vi "StartOrEnd.vi"(5 "Invert?":bool, 7 "StartOrEnd":string(combo), 10 "y":string, 11 "x":string) -> (2 "Equal?":bool)   [LabVIEW 2018]
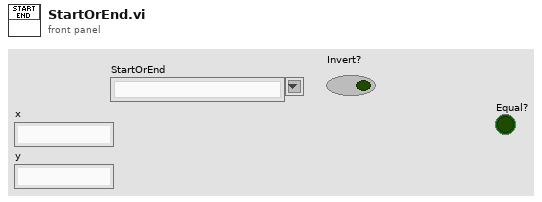
[diagram p1: front panel]
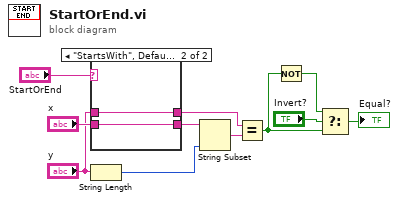
[diagram p0: block diagram]
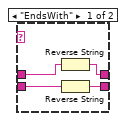
[diagram p2: hidden frame]
diagram:
  n1 = case shown="\"StartsWith\", Default" "StartOrEnd" {
    tunnel: [w14 w17] -> w5
    tunnel: "x" -> [w15 w17]
    tunnel: [w12 w16] -> w3
    tunnel: "y" -> [w13 w16]
    frame "EndsWith" {
      n2 = Reverse String(1:w13) -> (0:w12:string)
      n3 = Reverse String(1:w15) -> (0:w14:string)
    }
    frame "StartsWith", Default {
    }
  }
  n4 = String Length(string="y") -> (length=w4:i32)
  n5 = String Subset(string=w5, length (rest)=w4) -> (substring=w2:string)  [unwired: 1 in]
  n6 = Equal?(x=w3, y=w2) -> (x = y?=w1:bool)
  n7 = Not(x=w1) -> (.not. x?=w10:bool)
  n8 = Select(t=w10, s="Invert?", f=w1) -> (s? t:f=→"Equal?":bool)
